vi "WRITECSV (SubVI).vi"(10 "DATA PANEL":T1, 11 "PROCESS":string) -> ()   [LabVIEW 2021]
uses:
  <vilib>/Utility/file.llb/Write Delimited Spreadsheet (string).vi
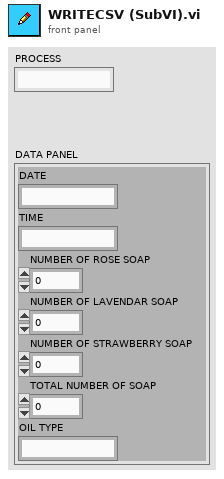
[diagram p1: front panel]
types:
  T1 = cluster{"DATE":string, "TIME":string, "NUMBER OF ROSE SOAP":dbl, "NUMBER OF LAVENDAR SOAP":dbl, "NUMBER OF STRAWBERRY SOAP":dbl, "TOTAL NUMBER OF SOAP":dbl, "OIL TYPE":string}
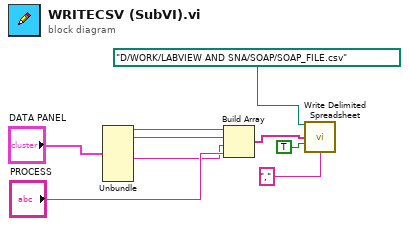
[diagram p0: block diagram]
diagram:
  n1 = Unbundle("DATA PANEL") -> ("DATE"=w4:string, "TIME"=w3:string, "OIL TYPE"=w8:string)  [unwired: 4 out]
  n2 = Build Array(w4, w3, w8, "PROCESS") -> (w1:string[])
  n3 = call-poly <vilib>:"Write Delimited Spreadsheet.vi"("file path (dialog if empty)"=path "D:/WORK/LABVIEW AND SNA/SOAP/SOAP_FILE.csv", "1D data"=w1, "append to file? (new file:F)"=TRUE, "delimiter (\\t)"="," ("delimiter (\\t)")) -> ()  [unwired: 10 in, 2 out]
